vi "Upload HEX File.vi"(0 "ChipKit Configuration":T1={"COM Port"="COM5", "Board Type"=enum."ChipKit Uno32", "Connection Type"=enum."USB / Serial", "Baud Rate (115200)"=115200, "Bytes Per Packet (15)"=15, "DI Port Num Pins"=0, "DO Port Num Pins"=0}, 2 "working directory":path=path "C:/Program Files (x86)/National Instruments/LabVIEW 2011/vi.lib/LabVIEW Hacker/LINX/Firmware/Tools/AVRDUDE", 3 "error in (no error)":errorcluster) -> (7 "ChipKit Configuration Out":T1={"COM Port"="", "Board Type"=enum."ChipKit Uno32", "Connection Type"=enum."USB / Serial", "Baud Rate (115200)"=115200, "Bytes Per Packet (15)"=15, "DI Port Num Pins"=0, "DO Port Num Pins"=0}, 10 "error out":errorcluster)   [LabVIEW 2011]
uses:
  <vilib>/LabVIEW Interface for ChipKit/Private/Type Defs/Board Type.ctl
  <vilib>/LabVIEW Interface for ChipKit/Private/Type Defs/Connection Type.ctl
  <vilib>/LabVIEW Interface for ChipKit/Private/Type Defs/Chipkit Resource.ctl
panel:
  out "concatenated string":string
  out "standard error":string
  out "standard output":string
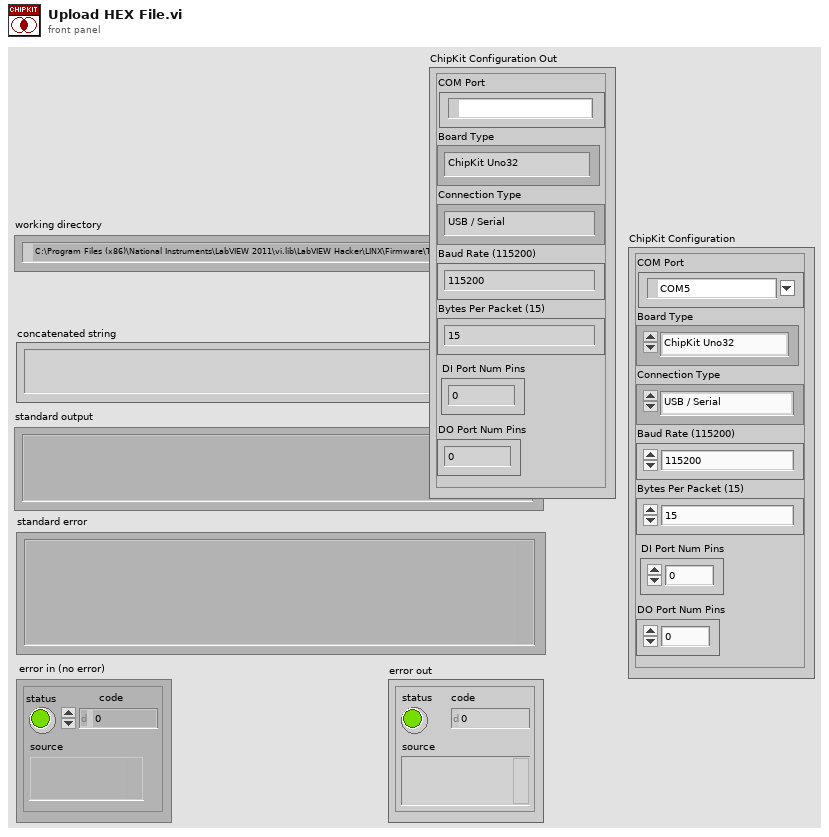
[diagram p1: front panel]
types:
  T1 = typedef "LabVIEW Interface for ChipKit.lvlib/Chipkit Resource.ctl" = cluster{"COM Port":refnum<visa-resource-name>, "Board Type":T2, "Connection Type":T3, "Baud Rate (115200)":u32, "Bytes Per Packet (15)":u32, "DI Port Num Pins":i32, "DO Port Num Pins":i32}
  T2 = typedef "LabVIEW Interface for ChipKit.lvlib/Board Type.ctl" = enum16{"ChipKit uC32", "ChipKit Uno32", "ChipKit Max32"}
  T3 = typedef "LabVIEW Interface for ChipKit.lvlib/Connection Type.ctl" = enum8{"USB / Serial", "XBEE", "BlueSmirf (Bluetooth)"}
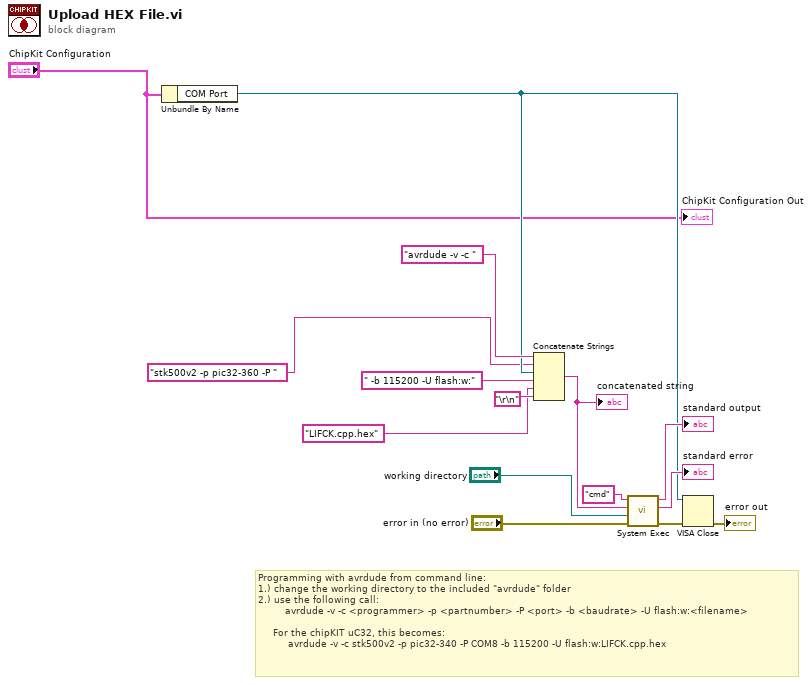
[diagram p0: block diagram]
diagram:
  # "Programming with avrdude from command line:\n1.) change the working directory to the included \"avrdude\" folder\n2.) use the following call:\n         avrdude -v -c <programmer> -p <partnumber> -P <port> -b <baudrate> -U flash:w:<filename>\n\n     For the chipKIT uC32, this becomes:     \n          avrdude -v -c stk500v2 -p pic32-340 -P COM8 -b 115200 -U flash:w:LIFCK.cpp.hex"
  n1 = Unbundle By Name("ChipKit Configuration") -> ("COM Port"=w4:refnum<visa-resource-name>)
  n2 = Concatenate Strings("avrdude -v -c " ("string"), "stk500v2 -p pic32-360 -P " ("string"), w4, " -b 115200 -U flash:w:" ("string"), "LIFCK.cpp.hex", "\r\n") -> (w5:string)
  "concatenated string" <- w5
  n3 = call <vilib>:"System Exec.vi"("error in (no error)"="error in (no error)", "working directory"="working directory", "standard input"=w5, "command line"="cmd") -> ("error out"=w11:errorcluster, "standard error"=→"standard error":string, "standard output"=→"standard output":string)  [unwired: 4 in, 1 out]
  n4 = VISA Close(VISA resource name=w4, error in (no error)=w11) -> (error out=→"error out":errorcluster)
  "ChipKit Configuration Out" <- "ChipKit Configuration"
